vi "Read Configured.vi"(8 "error in (no error)":errorcluster, 11 "Log Producer in":refnum<class "Log Producer.lvclass">) -> (0 "error out":errorcluster, 2 "Configured":bool, 3 "Log Producer out":refnum<class "Log Producer.lvclass">)   [LabVIEW 2020, in "AIM MIL-STD-1553 Engine.lvlib" / "Implementation.lvlib" / "Word Logging.lvlib" / "Log Producer.lvclass"]
uses:
  Log Producer.lvclass
  Log Producer.lvclass/Log Producer.ctl
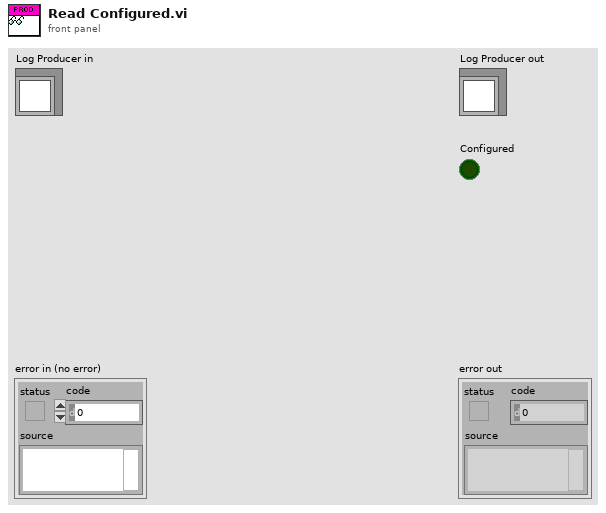
[diagram p1: front panel]
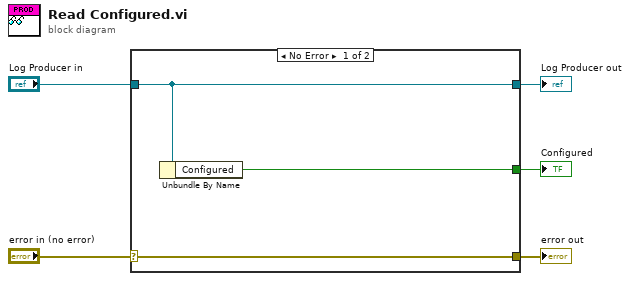
[diagram p0: block diagram]
diagram:
  n1 = case shown="No Error" "error in (no error)" {
    selector: "error in (no error)" -> [w8 w9]
    tunnel: [w8 w9] -> w4
    tunnel: [w7 w10] -> w2
    tunnel: "Log Producer in" -> [w7 w10]
    tunnel: [w6 _] -> w1
    frame No Error {
      n2 = Unbundle By Name(w7) -> ("Configured"=w6:bool)
    }
    frame Error {
    }
  }
  "error out" <- w4
  "Log Producer out" <- w2
  "Configured" <- w1
